vi "O_Data_to_Excel.vi"(8 "error in (no error)":errorcluster, 9 "ALL RESULT Array":dbl[][](array[numeric]) format="%_9g", 10 "REQUEST #":string, 11 "PROJECT #":string) -> (0 "error out":errorcluster)   [LabVIEW 2020]
uses:
  <vilib>/Utility/NIReport.llb/Report Type.ctl
  <vilib>/addons/_office/excel.llb/Excel Easy Table (num).vi
  <vilib>/Utility/NIReport.llb/NI_report.lvclass
  <vilib>/addons/_office/NI_ReportGenerationToolkit.lvlib
  <vilib>/Utility/NIReport.llb/Excel/NI_Excel.lvclass
  <vilib>/Utility/NIReport.llb/NI_ReportGenerationCore.lvlib
panel:
  # "Column 17"
  # "Column 18"
  # "Column 19"
  # "Column 20"
  # "Column 21"
  # "Column 22"
  # "Column 23"
  # "Column 24"
  # "Column 7"
  # "Column 8"
  # "Column 9"
  # "Column 10"
  # "Column 11"
  # "Column 12"
  # "Column 13"
  # "Column 14"
  # "Column 15"
  # "Column 16"
  # "Column 2"
  # "Column 3"
  # "Column 4"
  # "Column 5"
  # "Column 6"
  # "Column 0"
  # "Column 1"
  # "----------------Already Calculated---------------------"
  # "Tdon\n(ns)"
  # "Tr\n(ns)"
  # "Tdoff\n(ns)"
  # "Tf\n(ns)"
  # "on\ndi (A)"
  # "on\ndt (ns)"
  # "off\ndi (A)"
  # "off\ndt (ns)"
  # "on\ndv (V)"
  # "on\ndt (ns)"
  # "off\ndv (V)"
  # "off\ndt (ns)"
  # "Eon\n(uj)"
  # "Eoff\n(uj)"
  # "di/dt (on)\nA/us"
  # "di/dt (off)\nA/us"
  # "dv/dt (on)\nV/us"
  # "dv/dt (off)\nV/us"
  # "NULL\n(Separator)"
  # "Vce"
  # "Ice"
  # "Vge"
  # "Rg"
  # "Temperature"
  # "DUT  #"
  # "TEST #"
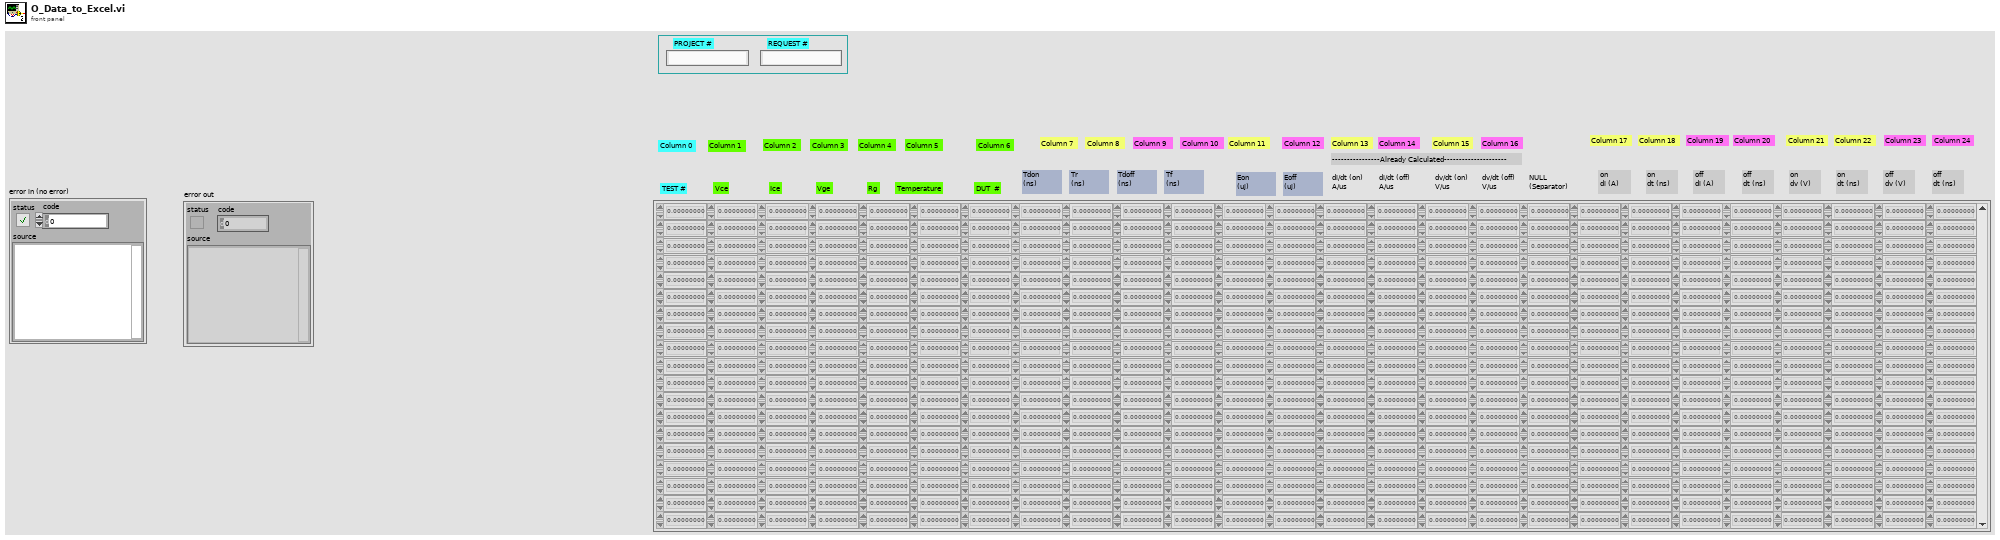
[diagram p1: front panel]
types:
  T1 = typedef "NI_ReportGenerationCore.lvlib/Report Type.ctl" = enum16{"HTML", "Word", "Excel"}
  T2 = enum16{"maximized", "minimized", "normal", "no change"}
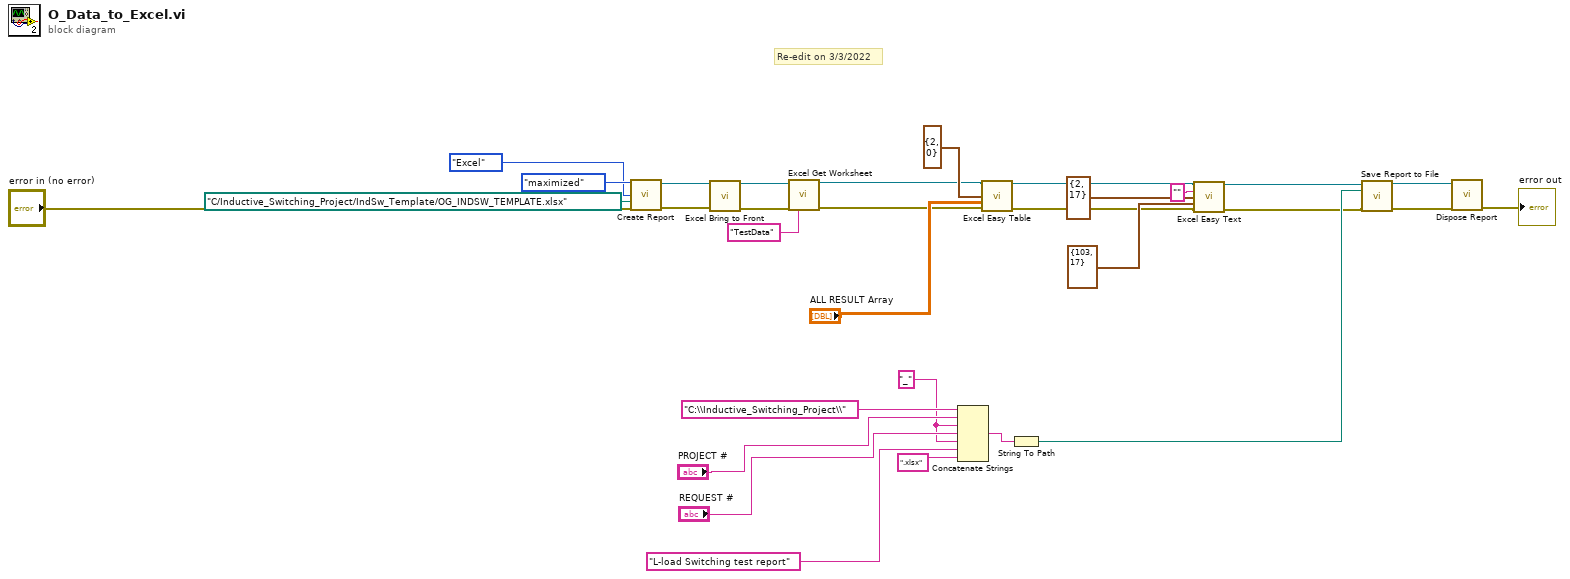
[diagram p0: block diagram]
diagram:
  w13 = "_" ("string")
  # "Re-edit on 3/3/2022"
  n1 = call <vilib>:"Create Report.vi"("window state (normal)"=T2."maximized", "report type"=Report_Type."Excel", "template (empty)"=path "C:/Inductive_Switching_Project/IndSw_Template/OG_INDSW_TEMPLATE.xlsx", "error in (no error)"="error in (no error)") -> ("report out"=w9:refnum<class "NI_report.lvclass">, "error out"=w11:errorcluster)  [unwired: 10 in]
  n2 = call <vilib>:"Excel Bring to Front.vi"("report in"=w9, "error in (no error)"=w11) -> ("report out"=w8:refnum<class "NI_report.lvclass">, "error out"=w10:errorcluster)  [unwired: 12 in]
  n3 = call <vilib>:"Excel Get Worksheet.vi"("report in"=w8, "error in (no error)"=w10, "name (\"\")"="TestData" ("name (\"\")")) -> ("report out"=w20:refnum<class "NI_report.lvclass">, "error out"=w21:errorcluster)  [unwired: 11 in]
  n4 = Concatenate Strings("C:\\Inductive_Switching_Project\\" ("string"), "PROJECT #", w13, "REQUEST #", w13, "L-load Switching test report" ("string"), ".xlsx" ("string")) -> (w31:string)
  n5 = call-poly <vilib>:"Excel Easy Table.vi"("report in"=w20, "start (0, 0)"=cluster{"row":i32, "column":i32} {"row"=2, "column"=0}, "text data"="ALL RESULT Array", "error in (no error)"=w21) -> ("report out"=w2:refnum<class "NI_report.lvclass">, "error out"=w4:errorcluster)  [unwired: 7 in, 3 out]
  n6 = String To Path(string=w31) -> (path=w19:path)
  n7 = call <vilib>:"Excel Easy Text.vi"("report in"=w2, "text"="", "start (-1, -1)"=cluster{"row":i32, "column":i32} {"row"=2, "column"=17}, "end (-1, -1)"=cluster{"row":i32, "column":i32} {"row"=103, "column"=17}, "error in (no error)"=w4) -> ("report out"=w1:refnum<class "NI_report.lvclass">, "error out"=w3:errorcluster)  [unwired: 6 in, 3 out]
  n8 = call-dynamic "Save Report to File.vi"("report in"=w1, "report file path"=w19, "error in (no error)"=w3) -> ("report out"=w17:refnum<class "NI_report.lvclass">, "error out"=w18:errorcluster)  [unwired: 11 in]
  n9 = call-dynamic "Dispose Report.vi"("report in"=w17, "error in (no error)"=w18) -> ("error out"=→"error out":errorcluster)  [unwired: 13 in]
